vi "Decoding.vi"(0 "Inputs-statusword":u16, 1 "Input-modes_of_operation_display":i8) -> (17 "Statusword_out":bool[](array[boolean]), 18 "Status":T1, 19 "Mode_of_operation":T2(ring))   [LabVIEW 2020]
uses:
  Statusword_status.ctl
  ElementDTD.lvlib
panel:
  out "Bit 7: waring":u16
  out "Bit 15:free":u16
  out "Bit 14:free":u16
  out "Bit 13:(following error)":u16
  out "Bit 12: (set_point_acknowledge)":u16
  out "Bit 11:internal_limit_active":u16
  out "Bit 10: target_reached":u16
  out "Bit 9 remote":u16
  out "Bit 8: dive is moving":u16
  out "Bit 6":u16
  out "Bit 5:quick_stop":u16
  out "Bit  4 Voltage_enabled":u16
  out "Bit 0 -  6 Regler Zustand":u16
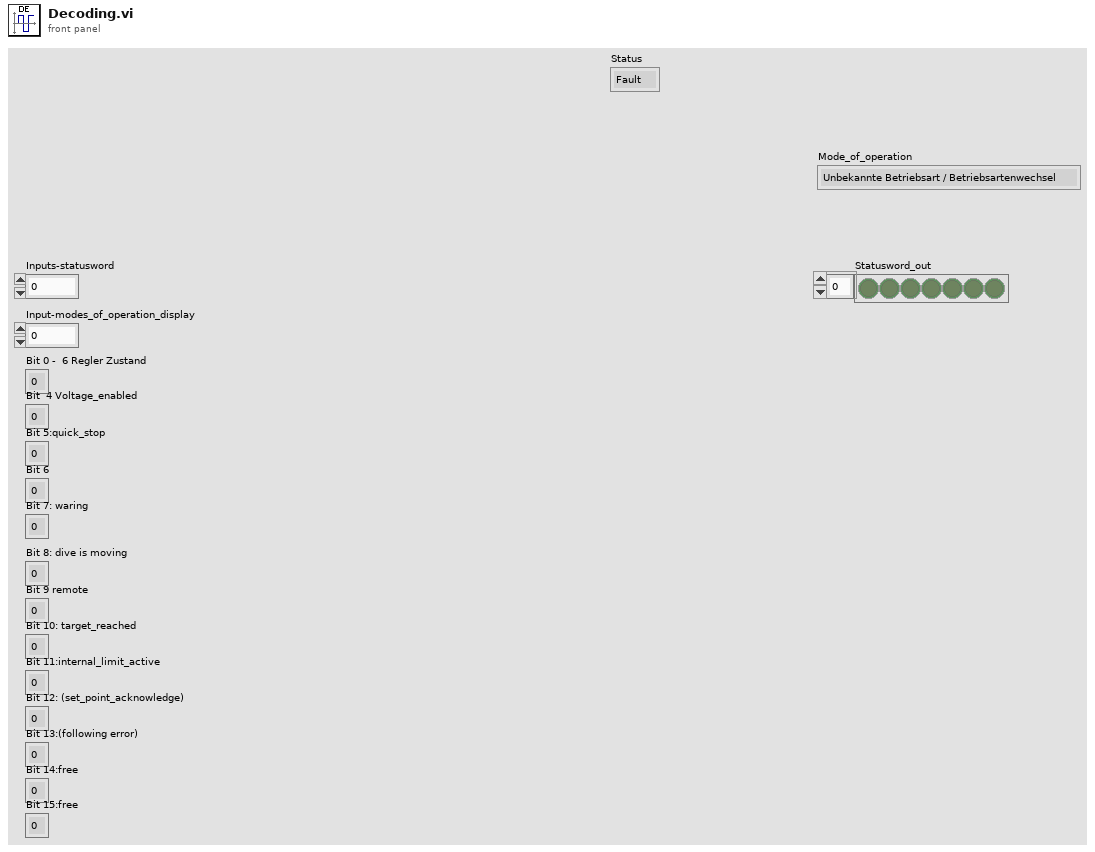
[diagram p1: front panel]
types:
  T1 = typedef "ElementDTD.lvlib/Statusword_status.ctl" = enum16{"Fault", "NOT_READY_TO_SWITCH_ON", "SWITCH_ON_DISABLED", "READY_TO_SWITCH_ON", "SWITCHED_ON", "OPERATION_ENABLE", "QUICK_STOP_ACTIVE"}
  T2 = enum16{"Unbekannte Betriebsart / Betriebsartenwechsel", "User_position_mode", "User_velocity_mode", "User_torque_mode", "Profile_position_mode", "Profile_velocity_mode", "Torque_profile_mode", "Homing_Mode", "Interpolated_position_mode"}
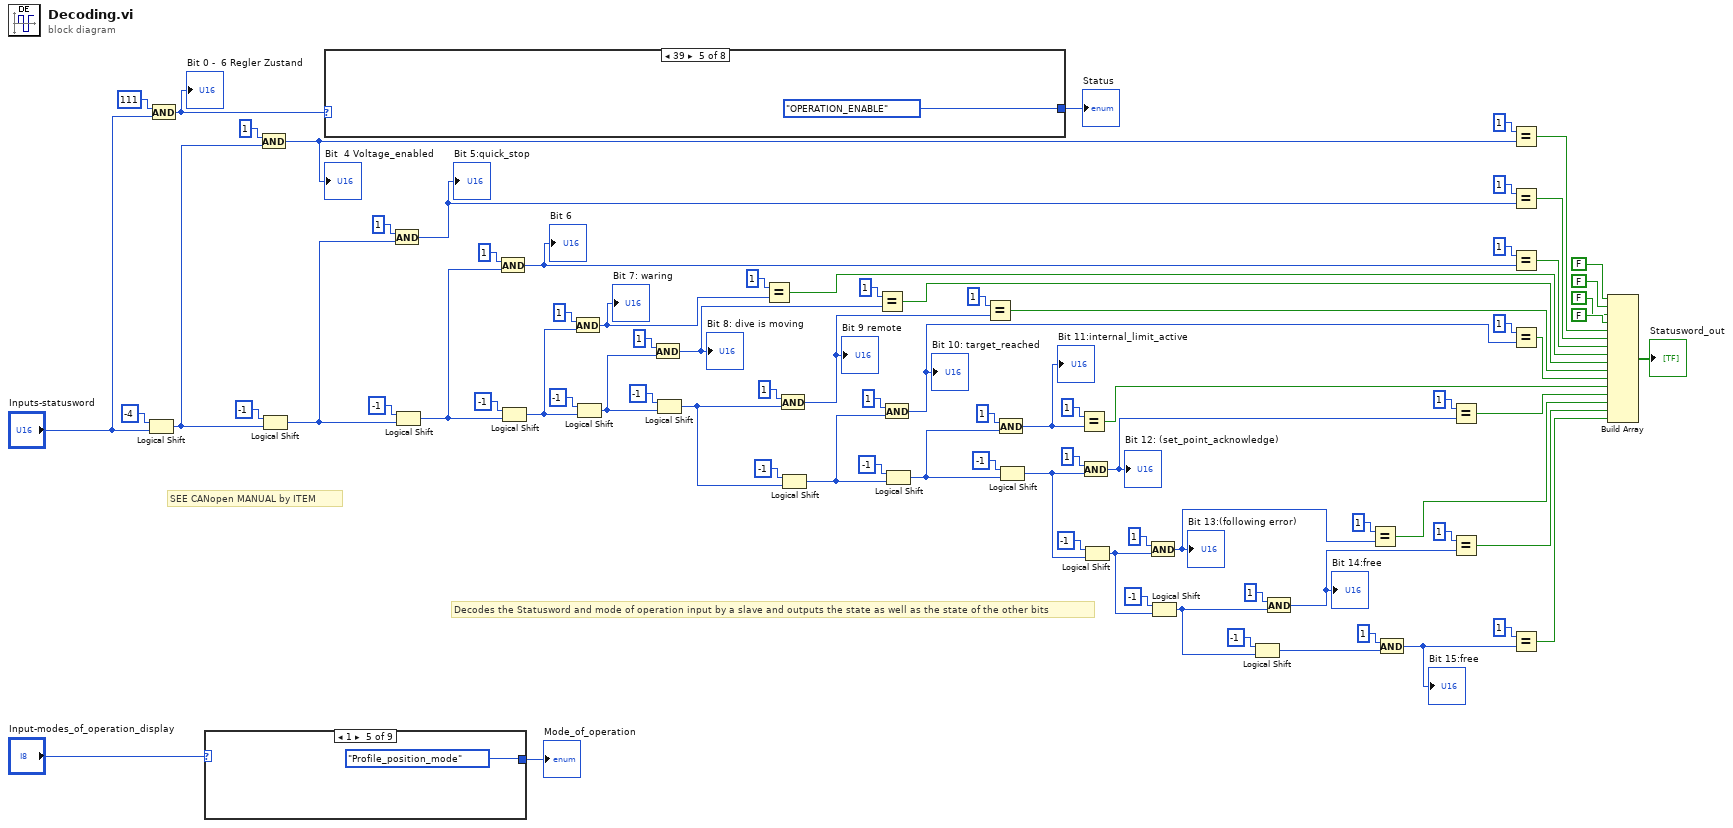
[diagram p0: block diagram]
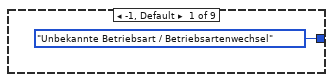
[diagram p2: hidden frame]
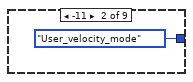
[diagram p3: hidden frame]
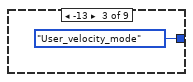
[diagram p4: hidden frame]
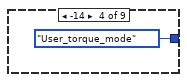
[diagram p5: hidden frame]
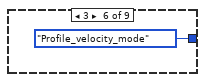
[diagram p6: hidden frame]
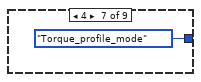
[diagram p7: hidden frame]
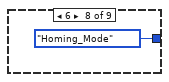
[diagram p8: hidden frame]
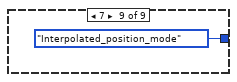
[diagram p9: hidden frame]
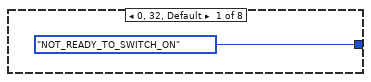
[diagram p10: hidden frame]
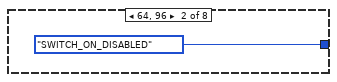
[diagram p11: hidden frame]
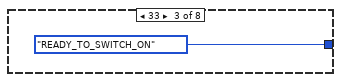
[diagram p12: hidden frame]
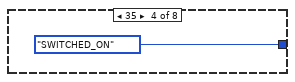
[diagram p13: hidden frame]
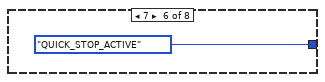
[diagram p14: hidden frame]
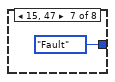
[diagram p15: hidden frame]
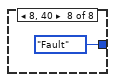
[diagram p16: hidden frame]
diagram:
  # "SEE CANopen MANUAL by ITEM"
  # "Decodes the Statusword and mode of operation input by a slave and outputs the state as well as the state of the other bits"
  n1 = Logical Shift(y=i16 -4, x="Inputs-statusword") -> (x << y=w79:u16)
  n2 = And(x=u16 111 ("Inputs-statusword"), y="Inputs-statusword") -> (x .and. y?=w4:u16)
  "Bit 0 -  6 Regler Zustand" <- w4
  n3 = case shown="1" "Input-modes_of_operation_display" {
    tunnel: [T2."Unbekannte Betriebsart / Betriebsartenwechsel" T2."User_velocity_mode" T2."User_velocity_mode" T2."User_torque_mode" T2."Profile_position_mode" T2."Profile_velocity_mode" T2."Torque_profile_mode" T2."Homing_Mode" T2."Interpolated_position_mode"] -> w2
    frame -1, Default {
    }
    frame -11 {
    }
    frame -13 {
    }
    frame -14 {
    }
    frame 1 {
    }
    frame 3 {
    }
    frame 4 {
    }
    frame 6 {
    }
    frame 7 {
    }
  }
  "Mode_of_operation" <- w2
  n4 = And(x=u16 1 ("Inputs-statusword"), y=w79) -> (x .and. y?=w27:u16)
  "Bit  4 Voltage_enabled" <- w27
  n5 = Logical Shift(y=i16 -1, x=w79) -> (x << y=w81:u16)
  n6 = case shown="39" w4 {
    tunnel: [Statusword_status."NOT_READY_TO_SWITCH_ON" Statusword_status."SWITCH_ON_DISABLED" Statusword_status."READY_TO_SWITCH_ON" Statusword_status."SWITCHED_ON" Statusword_status."OPERATION_ENABLE" Statusword_status."QUICK_STOP_ACTIVE" Statusword_status."Fault" Statusword_status."Fault"] -> w1
    frame 0, 32, Default {
    }
    frame 64, 96 {
    }
    frame 33 {
    }
    frame 35 {
    }
    frame 39 {
    }
    frame 7 {
    }
    frame 15, 47 {
    }
    frame 8, 40 {
    }
  }
  "Status" <- w1
  n7 = And(x=u16 1 ("Inputs-statusword"), y=w81) -> (x .and. y?=w28:u16)
  "Bit 5:quick_stop" <- w28
  n8 = Logical Shift(y=i16 -1, x=w81) -> (x << y=w77:u16)
  n9 = And(x=u16 1 ("Inputs-statusword"), y=w77) -> (x .and. y?=w29:u16)
  "Bit 6" <- w29
  n10 = Logical Shift(y=i16 -1, x=w77) -> (x << y=w75:u16)
  n11 = And(x=u16 1 ("Inputs-statusword"), y=w75) -> (x .and. y?=w40:u16)
  "Bit 7: waring" <- w40
  n12 = Logical Shift(y=i16 -1, x=w75) -> (x << y=w73:u16)
  n13 = And(x=u16 1 ("Inputs-statusword"), y=w73) -> (x .and. y?=w39:u16)
  "Bit 8: dive is moving" <- w39
  n14 = Logical Shift(y=i16 -1, x=w73) -> (x << y=w71:u16)
  n15 = Equal?(x=u16 1, y=w40) -> (x = y?=w33:bool)
  n16 = And(x=u16 1 ("Inputs-statusword"), y=w71) -> (x .and. y?=w38:u16)
  "Bit 9 remote" <- w38
  n17 = Logical Shift(y=i16 -1, x=w71) -> (x << y=w68:u16)
  n18 = Equal?(x=u16 1, y=w39) -> (x = y?=w34:bool)
  n19 = And(x=u16 1 ("Inputs-statusword"), y=w68) -> (x .and. y?=w37:u16)
  "Bit 10: target_reached" <- w37
  n20 = Logical Shift(y=i16 -1, x=w68) -> (x << y=w61:u16)
  n21 = Equal?(x=u16 1, y=w38) -> (x = y?=w35:bool)
  n22 = And(x=u16 1 ("Inputs-statusword"), y=w61) -> (x .and. y?=w46:u16)
  "Bit 11:internal_limit_active" <- w46
  n23 = Logical Shift(y=i16 -1, x=w61) -> (x << y=w9:u16)
  n24 = Equal?(x=u16 1, y=w46) -> (x = y?=w45:bool)
  n25 = And(x=u16 1 ("Inputs-statusword"), y=w9) -> (x .and. y?=w49:u16)
  "Bit 12: (set_point_acknowledge)" <- w49
  n26 = Logical Shift(y=i16 -1, x=w9) -> (x << y=w65:u16)
  n27 = And(x=u16 1 ("Inputs-statusword"), y=w65) -> (x .and. y?=w52:u16)
  "Bit 13:(following error)" <- w52
  n28 = Logical Shift(y=i16 -1, x=w65) -> (x << y=w62:u16)
  n29 = Logical Shift(y=i16 -1, x=w62) -> (x << y=w63:u16)
  n30 = And(x=u16 1 ("Inputs-statusword"), y=w62) -> (x .and. y?=w55:u16)
  "Bit 14:free" <- w55
  n31 = Equal?(x=u16 1, y=w52) -> (x = y?=w51:bool)
  n32 = And(x=u16 1 ("Inputs-statusword"), y=w63) -> (x .and. y?=w59:u16)
  "Bit 15:free" <- w59
  n33 = Equal?(x=u16 1, y=w49) -> (x = y?=w48:bool)
  n34 = Equal?(x=u16 1, y=w55) -> (x = y?=w54:bool)
  n35 = Equal?(x=u16 1, y=w27) -> (x = y?=w24:bool)
  n36 = Equal?(x=u16 1, y=w28) -> (x = y?=w25:bool)
  n37 = Equal?(x=u16 1, y=w29) -> (x = y?=w26:bool)
  n38 = Equal?(x=u16 1, y=w37) -> (x = y?=w36:bool)
  n39 = Equal?(x=u16 1, y=w59) -> (x = y?=w57:bool)
  n40 = Build Array(FALSE ("Element"), FALSE ("Element"), FALSE ("Element"), FALSE ("Element"), w24, w25, w26, w33, w34, w35, w36, w45, w48, w51, w54, w57) -> (→"Statusword_out":bool[])
